vi "Populate Symbol Map.vi"(8 "error in (no error)":errorcluster, 11 "TwinCAT ADS in":refnum<class "TwinCAT ADS.lvclass">) -> (0 "error out":errorcluster, 3 "TwinCAT ADS out":refnum<class "TwinCAT ADS.lvclass">)   [LabVIEW 2018, in "TwinCAT ADS.lvclass"]
uses:
  TwinCAT ADS.lvclass
  TwinCAT ADS.lvclass/TwinCAT ADS.ctl
  TwinCAT.Ads
  Get Symbol Map.vi
  <vilib>/Utility/error.llb/Trim Whitespace.vi
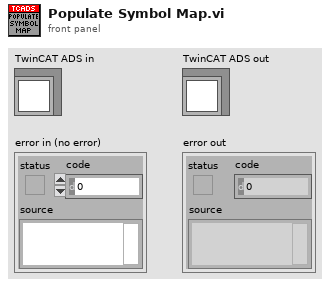
[diagram p1: front panel]
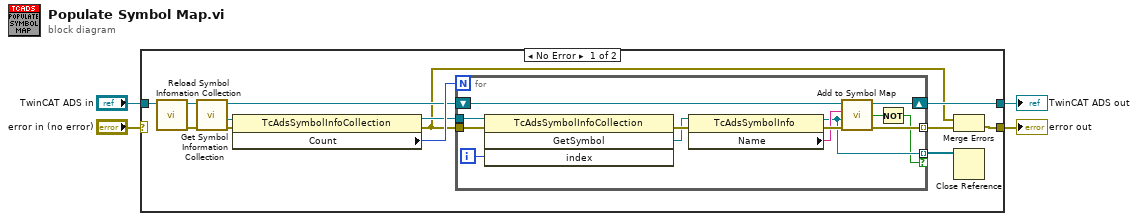
[diagram p0: block diagram]
diagram:
  n1 = case shown="No Error" "error in (no error)" {
    selector: "error in (no error)" -> [_ w32]
    tunnel: "TwinCAT ADS in" -> [w8 w31]
    tunnel: [w11 w32] -> w1
    tunnel: [w12 w31] -> w2
    frame No Error {
      n2 = call "Reload Symbol Infomation Collection.vi"("TwinCAT ADS in"=w8) -> ("error out"=w7:errorcluster, "TwinCAT ADS out"=w9:refnum<class "TwinCAT ADS.lvclass">)  [unwired: 9 in]
      n3 = call "Get Symbol Information Collection.vi"("error in (no error)"=w7, "TwinCAT ADS in"=w9) -> ("error out"=w15:errorcluster, ".NET AdsSymbolInfoCollection"=w14:refnum<k24>, "TwinCAT ADS out"=w13:refnum<class "TwinCAT ADS.lvclass">)  [unwired: 7 in]
      n4 = property class="TcAdsSymbolInfoCollection"(reference=w14, error in=w15) -> (reference out=w16:refnum<k24>, error out=w5:errorcluster, "Count"=w17:i32)
      n5 = for {
        N: w17 -> [_]
        tunnel: w16 -> [w29]
        tunnel: w5 -> [w30]
        shift-right: [w22] -> w12
        shift-left: w13 -> [w24]
        tunnel: [w21] -> w10 mode=indexing
        tunnel: [w20] -> w6 mode=indexing if=w18
        i -> [w26]
        n6 = invoke class="TcAdsSymbolInfoCollection" method="GetSymbol"(reference=w29, error in=w30, "index"=w26) -> (error out=w28:errorcluster, "GetSymbol"=w27:refnum<k24>)  [unwired: 1 in, 2 out]
        n7 = property class="TcAdsSymbolInfo"(reference=w27, error in=w28) -> (reference out=w20:refnum<k24>, error out=w25:errorcluster, "Name"=w23:string)
        n8 = call "Add to Symbol Map.vi"("error in (no error)"=w25, ".NET Symbol Information"=w20, "Symbol Name"=w23, "TwinCAT ADS in"=w24) -> ("error out"=w21:errorcluster, "Success?"=w19:bool, "TwinCAT ADS out"=w22:refnum<class "TwinCAT ADS.lvclass">)  [unwired: 5 in]
        n9 = Not(x=w19) -> (.not. x?=w18:bool)
      }
      n10 = Merge Errors(w5, w10) -> (w11:errorcluster)
      n11 = Close Reference(reference=w6) -> ()  [unwired: 1 in, 1 out]
    }
    frame Error {
    }
  }
  "error out" <- w1
  "TwinCAT ADS out" <- w2
